vi "Add Data Channels.vi"(8 "error in (no error)":errorcluster, 9 "progress queue":refnum<queue>, 10 "Framework Configuration":refnum<class "Framework Configuration.lvclass">, 11 "Item Ref in":T1 format="%.0x") -> (0 "error out":errorcluster, 3 "Item Ref out":T1 format="%.0x")   [LabVIEW 2017, in "DSF System Explorer.lvlib"]
uses:
  DSF System Explorer.lvlib
  <vilib>/NI Veristand/Custom Device API/Custom Device Item Ref.ctl
  progress window data.ctl
  DSF Core.lvlibp/Classes/Configuration/Core/Framework/Framework Configuration.lvclass
  <vilib>/NI Veristand/Custom Device API/Custom Device Channel Type.ctl
  <vilib>/NI Veristand/Custom Device API/Custom Device Channel.ctl
  Shared/Data Channel Page GUID.vi
  Shared/DSF Shared.lvlib
  DSF Core.lvlibp/Classes/Configuration/Core/Group/Group Configuration.lvclass
  DSF Core.lvlibp/Classes/Configuration/Core/Plugin/Plugin Configuration.lvclass
  DSF Core.lvlibp/Classes/Configuration/Core/Thread/Thread Configuration.lvclass
  DSF Core.lvlibp/Classes/Configuration/Core/Transfer/Transfer Configuration.lvclass
  DSF Core.lvlibp/Classes/Configuration/Core/Core Configuration.lvclass
  <vilib>/NI VeriStand/Custom Device API/Custom Device API.lvlib
  C:/Git/niveristand-data-sharing-framework-custom-device/VeriStand/Data Sharing Custom Device/Source/DSF Core.lvlibp/Classes/Configuration/Core/Core Configuration.lvclass
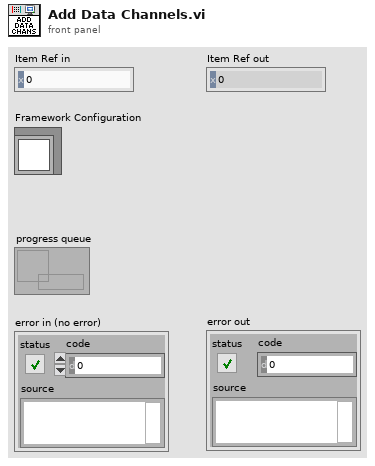
[diagram p1: front panel]
types:
  T1 = typedef "Custom Device API.lvlib/Custom Device Item Ref.ctl" = u64
  T2 = typedef "Custom Device API.lvlib/Custom Device Channel.ctl" = cluster{"Type":T3, "Units":string, "Default Value":dbl, "Faultable":bool, "Scalable":bool}
  T3 = typedef "Custom Device API.lvlib/Custom Device Channel Type.ctl" = enum16{"Input", "Output"}
  T4 = typedef "DSF Core.lvlibp/Plugin Configuration.lvclass/Core Plugin Configuration.ctl" = cluster{"name":string, "components":string[], "cycle timing":T5}
  T5 = typedef "DSF Core.lvlibp/DSF Timing Info.ctl" = cluster{"priority":u64, "decimation":u64, "offset":u64}
  T6 = typedef "DSF Core.lvlibp/DSF Settings Info.ctl" = cluster{"component":string, "values":cluster{"key":string, "value":string}[]}
  T7 = typedef "DSF Core.lvlibp/Thread Configuration.lvclass/Core Thread Configuration.ctl" = cluster{"processor":i32, "priority offset":i16}
  T8 = typedef "DSF Core.lvlibp/Group Configuration.lvclass/Core Group Configuration.ctl" = cluster{"name":string, "direction":T9, "cycle timing":T5, "timeout behavior":T10, "enable conversion":bool}
  T9 = typedef "DSF Core.lvlibp/DSF Direction.ctl" = enum8{"Tx", "Rx"}
  T10 = typedef "DSF Core.lvlibp/DSF Timeout Behavior.ctl" = enum8{"Increment Late Count", "Throw Error"}
  T11 = typedef "DSF Core.lvlibp/Transfer Configuration.lvclass/Core Transfer Configuration.ctl" = cluster{"name":string}
  T12 = typedef "DSF Core.lvlibp/Transfer Configuration.lvclass/Channel Configuration.ctl" = cluster{"configuration":T13, "component settings":T6[]}
  T13 = typedef "DSF Core.lvlibp/Channel Configuration.lvclass/Core Channel Configuration.ctl" = cluster{"name":string, "units":string, "engine data type":T14, "string data type":T14, "string offset":u64}
  T14 = typedef "DSF Core.lvlibp/DSF Data Type.ctl" = enum8{"Bool", "SGL", "DBL", "I8", "I16", "I32", "I64", "U8", "U16", "U32", "U64"}
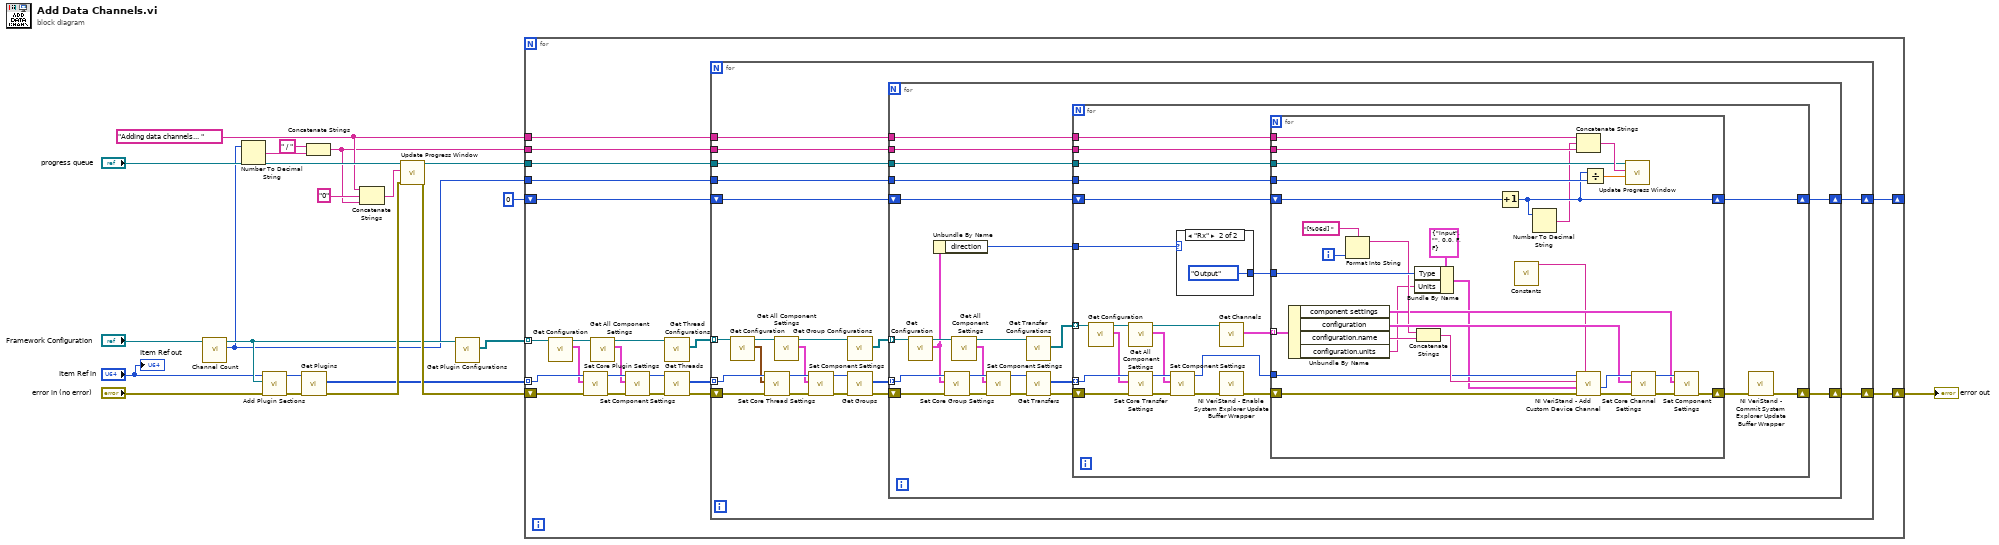
[diagram p0: block diagram]
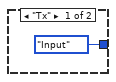
[diagram p2: hidden frame]
diagram:
  w12 = "Adding data channels... " ("message (\"\")")
  n1 = call-dynamic "Channel Count.vi"("Framework Configuration in"="Framework Configuration") -> ("channel count"=w3:i32, "Framework Configuration out"=w4:refnum<class "Framework Configuration.lvclass">)  [unwired: 8 in, 1 out]
  n2 = Number To Decimal String(number=w3) -> (decimal integer string=w16:string)  [unwired: 1 in]
  n3 = call "Add Plugin Sections.vi"("error in (no error)"="error in (no error)", "Framework Configuration"=w4, "Item Ref in"="Item Ref in") -> ("error out"=w19:errorcluster, "Item Ref out"=w18:T1)  [unwired: 7 in]
  n4 = call "Get Plugins.vi"("error in (no error)"=w19, "Item Ref in"=w18) -> ("error out"=w9:errorcluster, "Plugin refs"=w8:T1[])  [unwired: 7 in, 1 out]
  n5 = Concatenate Strings(" / " ("string"), w16) -> (w11:string)
  n6 = Concatenate Strings(w12, "0" ("string"), w11) -> (w10:string)
  n7 = call "Update Progress Window.vi"("error in (no error)"=w9, "message (\"\")"=w10, "progress queue in"="progress queue") -> ("error out"=w21:errorcluster, "progress queue out"=w14:refnum<queue>)  [unwired: 7 in]
  n8 = call "Get Plugin Configurations.vi"("Framework Configuration in"=w4) -> ("Plugin Configurations"=w7:refnum<class "Plugin Configuration.lvclass">[])  [unwired: 8 in, 2 out]
  n9 = for {
    tunnel: w14 -> [w41]
    tunnel: w12 -> [w40]
    tunnel: w11 -> [w39]
    tunnel: w8 -> [w28] mode=indexing
    tunnel: w3 -> [w38]
    tunnel: w7 -> [w30] mode=indexing
    shift-right: [w42] -> w20
    shift-left: w21 -> [w29]
    shift-right: [w36] -> _
    shift-left: 0 ("channel count") -> [w37]
    n10 = call "Get Configuration.vi"("Core Plugins Configuration in"=w30) -> ("configuration"=w27:T4, "Core Plugins Configuration out"=w24:refnum<class "Plugin Configuration.lvclass">)  [unwired: 8 in, 1 out]
    n11 = call "Set Core Plugin Settings.vi"("error in (no error)"=w29, "plugin configuration"=w27, "Item Ref in"=w28) -> ("error out"=w26:errorcluster, "Item Ref out"=w25:T1)  [unwired: 7 in]
    n12 = call "Get All Component Settings.vi"("Runtime Configuration in"=w24) -> ("component settings"=w23:T6[], "Runtime Configuration out"=w22:refnum<class "Plugin Configuration.lvclass">)  [unwired: 8 in, 1 out]
    n13 = call "Set Component Settings.vi"("error in (no error)"=w26, "component settings"=w23, "Item Ref in"=w25) -> ("error out"=w31:errorcluster, "Item Ref out"=w32:T1)  [unwired: 7 in]
    n14 = call "Get Thread Configurations.vi"("Plugin Configuration in"=w22) -> ("Thread Configurations"=w35:refnum<class "Thread Configuration.lvclass">[])  [unwired: 8 in, 2 out]
    n15 = call "Get Threads.vi"("error in (no error)"=w31, "Item Ref in"=w32) -> ("error out"=w34:errorcluster, "Plugin refs"=w33:T1[])  [unwired: 7 in, 1 out]
    n16 = for {
      tunnel: w33 -> [w51] mode=indexing
      shift-right: [w55] -> w42
      shift-left: w34 -> [w52]
      tunnel: w41 -> [w61]
      tunnel: w39 -> [w60]
      shift-right: [w58] -> w36
      shift-left: w37 -> [w59]
      tunnel: w40 -> [w57]
      tunnel: w38 -> [w56]
      tunnel: w35 -> [w53] mode=indexing
      n17 = call "Get Configuration.vi"("Core Threads Configuration in"=w53) -> ("configuration"=w49:T7, "Core Threads Configuration out"=w50:refnum<class "Thread Configuration.lvclass">)  [unwired: 8 in, 1 out]
      n18 = call "Set Core Thread Settings.vi"("error in (no error)"=w52, "thread configuration"=w49, "Item Ref in"=w51) -> ("error out"=w48:errorcluster, "Item Ref out"=w47:T1)  [unwired: 7 in]
      n19 = call "Get All Component Settings.vi"("Runtime Configuration in"=w50) -> ("component settings"=w43:T6[], "Runtime Configuration out"=w44:refnum<class "Thread Configuration.lvclass">)  [unwired: 8 in, 1 out]
      n20 = call "Set Component Settings.vi"("error in (no error)"=w48, "component settings"=w43, "Item Ref in"=w47) -> ("error out"=w45:errorcluster, "Item Ref out"=w46:T1)  [unwired: 7 in]
      n21 = call "Get Group Configurations.vi"("Thread Configuration in"=w44) -> ("Group Configurations"=w54:refnum<class "Group Configuration.lvclass">[])  [unwired: 8 in, 2 out]
      n22 = call "Get Groups.vi"("error in (no error)"=w45, "Plugin Ref in"=w46) -> ("error out"=w63:errorcluster, "Group refs"=w62:T1[])  [unwired: 7 in, 1 out]
      n23 = for {
        shift-right: [w77] -> w55
        shift-left: w63 -> [w74]
        tunnel: w62 -> [w73] mode=indexing
        tunnel: w54 -> [w68] mode=indexing
        tunnel: w61 -> [w83]
        tunnel: w60 -> [w81]
        shift-right: [w80] -> w58
        shift-left: w59 -> [w82]
        tunnel: w57 -> [w79]
        tunnel: w56 -> [w78]
        n24 = call "Get Configuration.vi"("Core Groups Configuration in"=w68) -> ("configuration"=w64:T8, "Core Groups Configuration out"=w67:refnum<class "Group Configuration.lvclass">)  [unwired: 8 in, 1 out]
        n25 = Unbundle By Name(w64) -> ("direction"=w75:T9)
        n26 = call "Set Core Group Settings.vi"("error in (no error)"=w74, "group configuration"=w64, "Item Ref in"=w73) -> ("error out"=w72:errorcluster, "Item Ref out"=w71:T1)  [unwired: 7 in]
        n27 = call "Get All Component Settings.vi"("Runtime Configuration in"=w67) -> ("component settings"=w66:T6[], "Runtime Configuration out"=w65:refnum<class "Group Configuration.lvclass">)  [unwired: 8 in, 1 out]
        n28 = call "Set Component Settings.vi"("error in (no error)"=w72, "component settings"=w66, "Item Ref in"=w71) -> ("error out"=w70:errorcluster, "Item Ref out"=w69:T1)  [unwired: 7 in]
        n29 = call "Get Transfer Configurations.vi"("Group Configuration in"=w65) -> ("Transfer Configurations"=w76:refnum<class "Transfer Configuration.lvclass">[])  [unwired: 8 in, 2 out]
        n30 = call "Get Transfers.vi"("error in (no error)"=w70, "Group Ref in"=w69) -> ("error out"=w85:errorcluster, "Transfer refs"=w84:T1[])  [unwired: 7 in, 1 out]
        n31 = for {
          shift-right: [w87] -> w77
          shift-left: w85 -> [w108]
          tunnel: w84 -> [w106] mode=indexing
          tunnel: w83 -> [w90]
          shift-right: [w86] -> w80
          shift-left: w82 -> [w88]
          tunnel: w81 -> [w91]
          tunnel: w79 -> [w92]
          tunnel: w78 -> [w89]
          tunnel: w75 -> [w95]
          tunnel: w76 -> [w107] mode=indexing
          n32 = call "Get Configuration.vi"("Core Transfers Configuration in"=w107) -> ("configuration"=w105:T11, "Core Transfers Configuration out"=w101:refnum<class "Transfer Configuration.lvclass">)  [unwired: 8 in, 1 out]
          n33 = call "Get All Component Settings.vi"("Runtime Configuration in"=w101) -> ("component settings"=w100:T6[], "Runtime Configuration out"=w99:refnum<class "Transfer Configuration.lvclass">)  [unwired: 8 in, 1 out]
          n34 = call "Set Core Transfer Settings.vi"("error in (no error)"=w108, "transfer configuration"=w105, "Item Ref in"=w106) -> ("error out"=w104:errorcluster, "Item Ref out"=w103:T1)  [unwired: 7 in]
          n35 = call "Set Component Settings.vi"("error in (no error)"=w104, "component settings"=w100, "Item Ref in"=w103) -> ("error out"=w102:errorcluster, "Item Ref out"=w94:T1)  [unwired: 7 in]
          n36 = case shown="\"Rx\"" w95 {
            tunnel: [Custom_Device_Channel_Type."Input" ("Type") Custom_Device_Channel_Type."Output" ("Type")] -> w98
            frame "Tx" {
            }
            frame "Rx" {
            }
          }
          n37 = call "Get Channels.vi"("Transfer Configuration in"=w99) -> ("channels"=w96:T12[])  [unwired: 8 in, 2 out]
          n38 = call "NI VeriStand - Enable System Explorer Update Buffer Wrapper.vi"("error in"=w102) -> ("error out"=w93:errorcluster)  [unwired: 10 in]
          n39 = for {
            tunnel: w94 -> [w133]
            tunnel: w98 -> [w136]
            tunnel: w96 -> [w130] mode=indexing
            shift-right: [w114] -> w97
            shift-left: w93 -> [w132]
            tunnel: w92 -> [w122]
            tunnel: w91 -> [w121]
            tunnel: w90 -> [w120]
            tunnel: w89 -> [w119]
            shift-right: [w117] -> w86
            shift-left: w88 -> [w118]
            i -> [w125]
            n40 = Unbundle By Name(w130) -> ("component settings"=w113:T6[], "configuration"=w128:T13, "configuration.name"=w127:string, "configuration.units"=w111:string)
            n41 = Format Into String(format string="[%06d] ", w125) -> (resulting string=w126:string)  [unwired: 2 in, 1 out]
            n42 = Bundle By Name(cluster=T2 {"Type"=enum."Input", "Units"="", "Default Value"=0.0, "Faultable"=FALSE, "Scalable"=FALSE} ("Channel"), "Type"=w136, "Units"=w111) -> (w112:T2)
            n43 = Concatenate Strings(w126, w127) -> (w135:string)
            n44 = Increment(x=w118) -> (x+1=w117:i32)
            n45 = call-poly "Constants.vi"() -> ("Status GUID"=w110:string)  [unwired: 11 in]
            n46 = Number To Decimal String(number=w117) -> (decimal integer string=w109:string)  [unwired: 1 in]
            n47 = Concatenate Strings(w122, w109, w121) -> (w124:string)
            n48 = call <vilib>:"NI VeriStand - Add Custom Device Channel.vi"("GUID (Default Channel)"=w110, "error in (no error)"=w132, "Channel"=w112, "Channel Name"=w135, "Parent Ref in"=w133) -> ("error out"=w131:errorcluster, "Channel Ref"=w129:T1)  [unwired: 3 in, 2 out]
            n49 = Divide(x=w117, y=w119) -> (x/y=w123:dbl)
            n50 = call "Update Progress Window.vi"("progress (0)"=w123, "message (\"\")"=w124, "progress queue in"=w120) -> ()  [unwired: 7 in, 2 out]
            n51 = call "Set Core Channel Settings.vi"("error in (no error)"=w131, "channel configuration"=w128, "Item Ref in"=w129) -> ("error out"=w116:errorcluster, "Item Ref out"=w115:T1)  [unwired: 7 in]
            n52 = call "Set Component Settings.vi"("error in (no error)"=w116, "component settings"=w113, "Item Ref in"=w115) -> ("error out"=w114:errorcluster)  [unwired: 7 in, 1 out]
          }
          n53 = call "NI VeriStand - Commit System Explorer Update Buffer Wrapper.vi"("error in"=w97) -> ("error out"=w87:errorcluster)  [unwired: 10 in]
        }
      }
    }
  }
  "error out" <- w20
  "Item Ref out" <- "Item Ref in"
